vi "DI Pulse Check.vi"(8 "Min Pulse Off Time [CAD]":sgl, 9 "Engine Speed [RPM]":sgl, 11 "DI Cluster":T1) -> (0 "DI Pulse Overlap Error":bool)   [LabVIEW 2015, in "ECS-RT.lvlib"]
uses:
  ECS-RT.lvlib
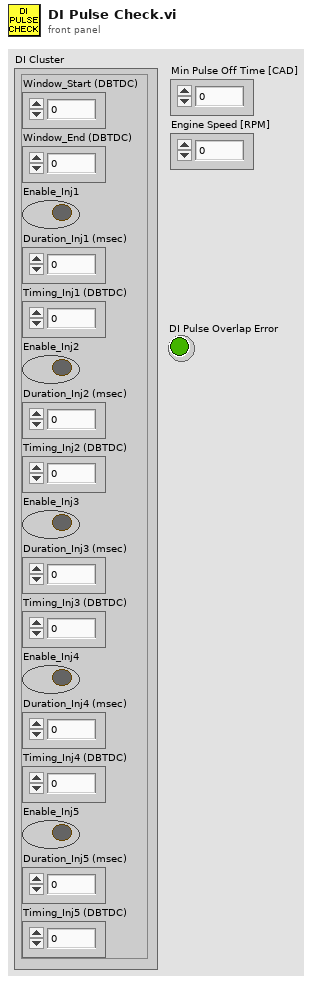
[diagram p1: front panel]
types:
  T1 = cluster{"Window_Start (DBTDC)":sgl, "Window_End (DBTDC)":sgl, "Enable_Inj1":bool, "Duration_Inj1 (msec)":sgl, "Timing_Inj1 (DBTDC)":sgl, "Enable_Inj2":bool, "Duration_Inj2 (msec)":sgl, "Timing_Inj2 (DBTDC)":sgl, "Enable_Inj3":bool, "Duration_Inj3 (msec)":sgl, "Timing_Inj3 (DBTDC)":sgl, "Enable_Inj4":bool, "Duration_Inj4 (msec)":sgl, "Timing_Inj4 (DBTDC)":sgl, "Enable_Inj5":bool, "Duration_Inj5 (msec)":sgl, "Timing_Inj5 (DBTDC)":sgl}
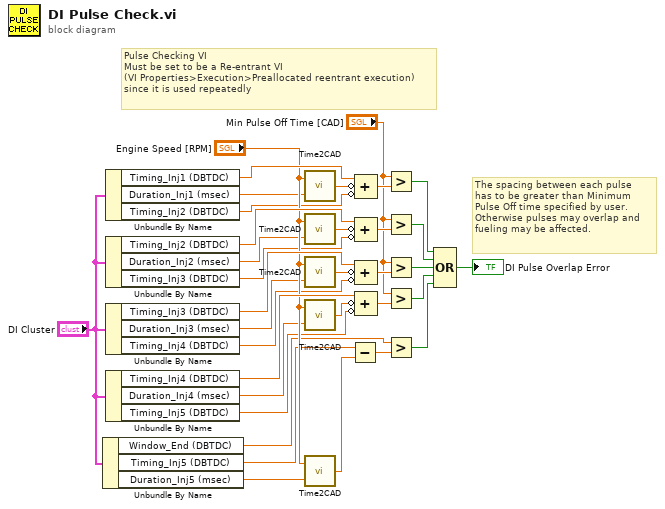
[diagram p0: block diagram]
diagram:
  # "Pulse Checking VI\nMust be set to be a Re-entrant VI \n(VI Properties>Execution>Preallocated reentrant execution)\nsince it is used repeatedly"
  # "The spacing between each pulse\nhas to be greater than Minimum \nPulse Off time specified by user.\nOtherwise pulses may overlap and\nfueling may be affected."
  n1 = Unbundle By Name("DI Cluster") -> ("Window_End (DBTDC)"=w1:sgl, "Timing_Inj5 (DBTDC)"=w19:sgl, "Duration_Inj5 (msec)"=w2:sgl)
  n2 = Unbundle By Name("DI Cluster") -> ("Timing_Inj1 (DBTDC)"=w34:sgl, "Duration_Inj1 (msec)"=w10:sgl, "Timing_Inj2 (DBTDC)"=w9:sgl)
  n3 = Unbundle By Name("DI Cluster") -> ("Timing_Inj2 (DBTDC)"=w29:sgl, "Duration_Inj2 (msec)"=w8:sgl, "Timing_Inj3 (DBTDC)"=w7:sgl)
  n4 = Unbundle By Name("DI Cluster") -> ("Timing_Inj3 (DBTDC)"=w23:sgl, "Duration_Inj3 (msec)"=w6:sgl, "Timing_Inj4 (DBTDC)"=w5:sgl)
  n5 = Unbundle By Name("DI Cluster") -> ("Timing_Inj4 (DBTDC)"=w24:sgl, "Duration_Inj4 (msec)"=w4:sgl, "Timing_Inj5 (DBTDC)"=w3:sgl)
  n6 = call <vilib>:"Time2CAD.vi"("Time [ms]"=w10, "Speed (RPM)"="Engine Speed [RPM]") -> ("CAD"=w33:sgl)
  n7 = call <vilib>:"Time2CAD.vi"("Time [ms]"=w8, "Speed (RPM)"="Engine Speed [RPM]") -> ("CAD"=w30:sgl)
  n8 = call <vilib>:"Time2CAD.vi"("Time [ms]"=w6, "Speed (RPM)"="Engine Speed [RPM]") -> ("CAD"=w28:sgl)
  n9 = call <vilib>:"Time2CAD.vi"("Time [ms]"=w4, "Speed (RPM)"="Engine Speed [RPM]") -> ("CAD"=w25:sgl)
  n10 = call <vilib>:"Time2CAD.vi"("Time [ms]"=w2, "Speed (RPM)"="Engine Speed [RPM]") -> ("CAD"=w20:sgl)
  n11 = Subtract(x=w19, y=w20) -> (x-y=w18:sgl)
  n12 = Compound Arithmetic op=ADD(w34, invert w33, invert w9) -> (w32:sgl)
  n13 = Compound Arithmetic op=ADD(w29, invert w30, invert w7) -> (w31:sgl)
  n14 = Compound Arithmetic op=ADD(w23, invert w28, invert w5) -> (w27:sgl)
  n15 = Compound Arithmetic op=ADD(w24, invert w25, invert w3) -> (w26:sgl)
  n16 = Greater?(x="Min Pulse Off Time [CAD]", y=w32) -> (0:w16:bool)
  n17 = Greater?(x="Min Pulse Off Time [CAD]", y=w31) -> (0:w15:bool)
  n18 = Greater?(x="Min Pulse Off Time [CAD]", y=w27) -> (0:w14:bool)
  n19 = Greater?(x="Min Pulse Off Time [CAD]", y=w26) -> (0:w13:bool)
  n20 = Greater?(x=w1, y=w18) -> (0:w12:bool)
  n21 = Compound Arithmetic op=OR(w16, w15, w14, w13, w12) -> (→"DI Pulse Overlap Error":bool)
